vi "to string.vi"(8 "error in":errorcluster, 11 "Submodule EOL configuration":refnum<class "Submodule EOL configuration.lvclass">) -> (0 "error out":errorcluster, 1 "data":string, 2 "version":string, 3 "Submodule EOL configuration out":refnum<class "Submodule EOL configuration.lvclass">)   [LabVIEW 2025, in "Submodule EOL.lvlib" / "Submodule EOL configuration.lvclass"]
doc: "Provides an interface for saving a module configuration to a file or other serialized data source. It is recommended that all children of this class store data in two sets--data required for its own initialization, and any data required for parent initialization--and that each implementation uses the <b>Call Parent Method</b> primitive to serialize parent information.Copyright 2017 National Instruments Corporation\n\nLicensed under the Apache License, Version 2.0 (the \"License\"); you may not use this file except in compliance with the License. You may obtain a copy of the License at http://www.apache.org/licenses/LICENSE-2.0\nUnless required by applicable law or agreed to in writing, software distributed under the License is distributed on an \"AS IS\" BASIS, WITHOUT WARRANTIES OR CONDITIONS OF ANY KIND, either express or implied. See the License for the specific language governing permissions and limitations under the License."
uses:
  Submodule EOL configuration.lvclass
  Submodule EOL configuration.lvclass/Submodule EOL configuration.ctl
  Users/Public/Documents/Sandia National Labs/TSS Plugin/CEF.lvlibp/serializable configuration/CEF_serializable configuration.lvclass
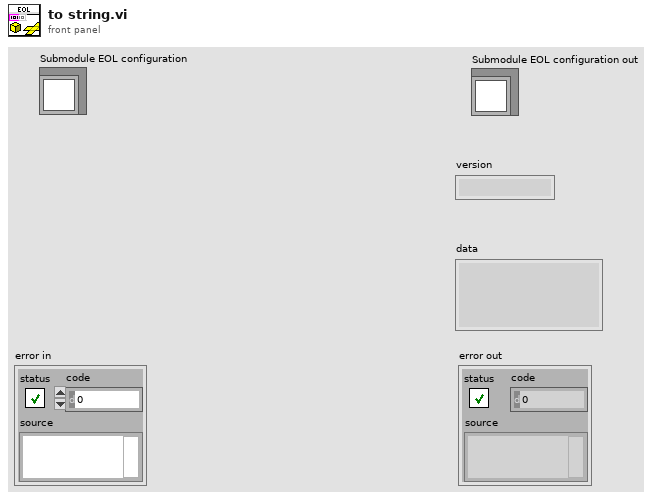
[diagram p1: front panel]
types:
  T1 = typedef "Submodule EOL configuration.lvclass/Submodule EOL.ctl" = cluster{"PLC Folder Names":string[][], "Timeout Connect OPC":dbl, "Connect OPC Trial":u32, "PLC URL":string, "Digitial IO":string, "HiPOT":string, "ACIR with Switch":string, "DMM with Switch":string, "Ignition Folder Names":string[][], "Ignition URL":string}
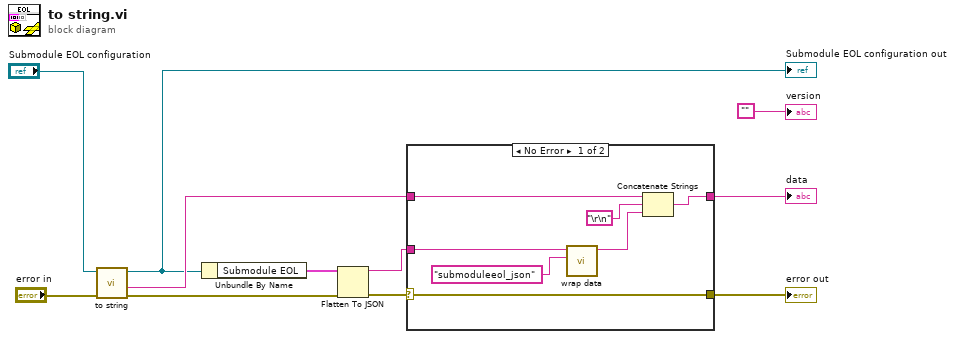
[diagram p0: block diagram]
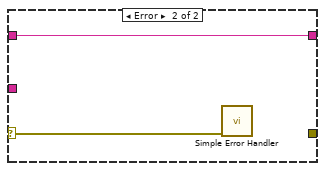
[diagram p2: hidden frame]
diagram:
  n1 = call-parent "to string.vi"("error in"="error in", "CEF_Configuration in"="Submodule EOL configuration") -> ("error out"=w9:errorcluster, "data"=w4:string, "CEF_Configuration out"=w1:refnum<class "Submodule EOL configuration.lvclass">)  [unwired: 6 in, 1 out]
  "Submodule EOL configuration out" <- w1
  n2 = Unbundle By Name(w1) -> ("Submodule EOL"=w10:T1)
  n3 = Flatten To JSON(anything=w10, error in (no error)=w9) -> (JSON string=w7:string, 11:w6:errorcluster)  [unwired: 1 in]
  n4 = case shown="No Error" w6 {
    selector: w6 -> [w18 w20]
    tunnel: [w18 _] -> w5
    tunnel: w7 -> [w16 _]
    tunnel: w4 -> [w15 w19]
    tunnel: [w13 w19] -> w3
    frame No Error {
      n5 = call "wrap data.vi"("identifier"="submoduleeol_json" ("additional identifier"), "data to wrap"=w16) -> ("wrapped data"=w17:string)  [unwired: 9 in]
      n6 = Concatenate Strings(w15, "\r\n", w17) -> (w13:string)
    }
    frame Error {
      n7 = call <vilib>:"Simple Error Handler.vi"("error in (no error)"=w20) -> ()  [unwired: 4 in, 5 out]
    }
  }
  "error out" <- w5
  "data" <- w3
  "version" <- ""
